vi "draw.vi"(0 "reference":refnum<class "Grid.lvclass">, 1 "graphics":refnum<class "Graphics.lvclass">, 2 "bounds":T1 {"height" format="%.2f"; "width" format="%.2f"; "y" format="%.2f"; "x" format="%.2f"}, 3 "ForceRedrawGrid":bool, 5 "error in (no error)":errorcluster) -> (14 "reference out":refnum<class "Grid.lvclass">, 19 "error out":errorcluster)   [LabVIEW 2016, in "Grid.lvclass"]
doc: "public void draw(Graphics2D g2, Rectangle2D bounds)"
uses:
  <resource>/Framework/Providers/Open_GDS/UML/Grid_class/Grid.lvclass
  <resource>/Framework/Providers/Open_GDS/UML/Graphics_class/Graphics.lvclass
  <resource>/Framework/Providers/Open_GDS/UML/General/Rectangle/Rectangle Rectangle2D.ctl
  <resource>/Framework/Providers/Open_GDS/UML/General/Point/Point Point2D.ctl
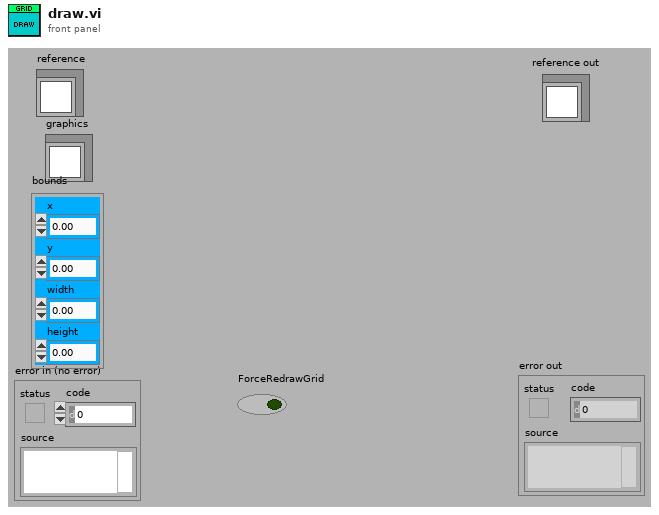
[diagram p1: front panel]
types:
  T1 = typedef "Rectangle Rectangle2D.ctl" = cluster{"x":dbl, "y":dbl, "width":dbl, "height":dbl}
  T2 = typedef "Point Point2D.ctl" = cluster{"x":dbl, "y":dbl}
  T3 = typedef "Grid.lvclass/ObjectAttributes.ctl" = cluster{"gridX":dbl, "gridY":dbl, "gridColor":u32}
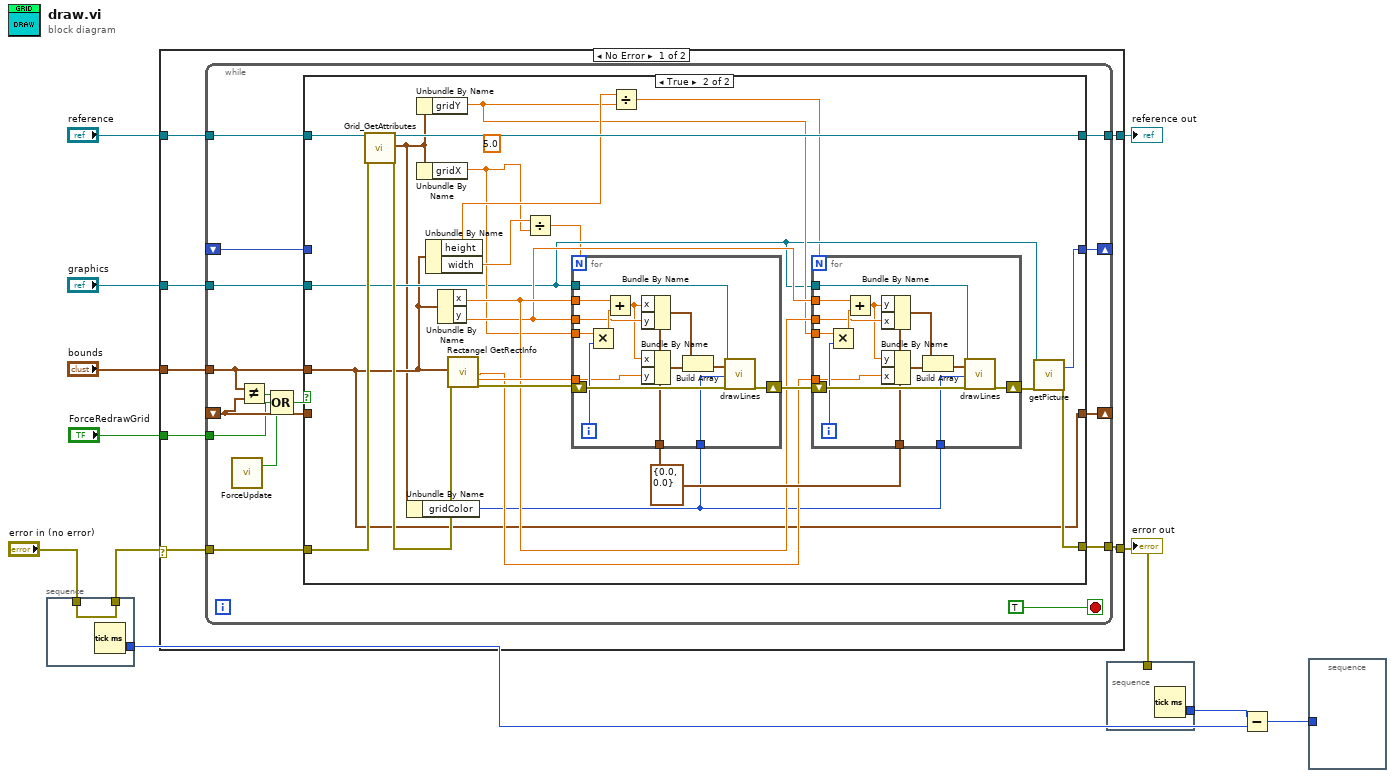
[diagram p0: block diagram]
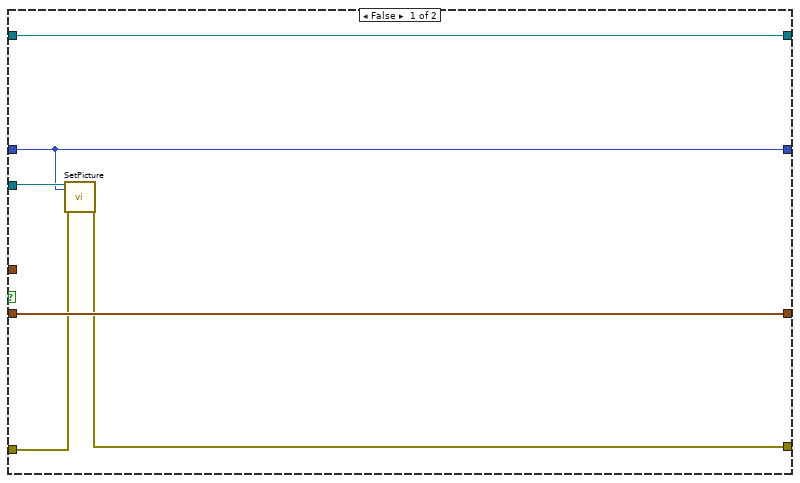
[diagram p2: hidden frame]
diagram:
  n1 = stacked-sequence {
    tunnel: [w13] -> w7
    tunnel: [w12] -> w5
    tunnel: "error in (no error)" -> [w12]
    frame #0 {
      n2 = Tick Count (ms)() -> (millisecond timer value=w13:u32)
    }
  }
  n3 = case shown="No Error" w5 {
    selector: w5 -> [w18 w96]
    tunnel: "reference" -> [w20 w97]
    tunnel: [w15 w96] -> w4
    tunnel: [w19 w97] -> w10
    tunnel: "bounds" -> [w16 _]
    tunnel: "graphics" -> [w17 _]
    tunnel: "ForceRedrawGrid" -> [w14 _]
    frame No Error {
      n4 = while {
        tunnel: w20 -> [w35]
        tunnel: [w34] -> w19
        tunnel: w18 -> [w33]
        tunnel: w17 -> [w32]
        tunnel: w16 -> [w27]
        tunnel: [w31] -> w15
        shift-right: [w29] -> _
        shift-left: _ -> [w28]
        shift-right: [w25] -> _
        shift-left: _ -> [w26]
        tunnel: w14 -> [w24]
        stop <- TRUE stop-if-true
        n5 = call <resource>:"ForceUpdate.vi"() -> ("Force"=w21:bool)  [unwired: 19 in]
        n6 = Not Equal?(x=w27, y=w28) -> (x != y?=w23:bool)
        n7 = Compound Arithmetic op=OR(w23, w24, w21) -> (w22:bool)
        n8 = case shown="True" w22 {
          tunnel: w35 -> [w40 w65]
          tunnel: [w40 w64] -> w34
          tunnel: w33 -> [w38 w63]
          tunnel: w32 -> [w39 w46]
          tunnel: w27 -> [_ w43]
          tunnel: [w37 w48] -> w31
          tunnel: [w41 w43] -> w29
          tunnel: w28 -> [w41 _]
          tunnel: w26 -> [w36 _]
          tunnel: [w36 w47] -> w25
          frame False {
            n9 = call-dynamic "SetPicture.vi"("reference"=w39, "picture"=w36, "error in (no error)"=w38) -> ("error out"=w37:errorcluster)  [unwired: 15 in, 1 out]
          }
          frame True {
            w56 = T2 {"x"=0.0, "y"=0.0} ("point2D")
            (unwired) 5.0 ("lower limit")
            n10 = call <resource>:"Grid_GetAttributes.vi"("reference in"=w65, "error in (no error)"=w63) -> ("reference out"=w64:refnum<class "Grid.lvclass">, "Data"=w42:T3, "error out"=w62:errorcluster)  [unwired: 1 in, 14 out]
            n11 = Unbundle By Name(w42) -> ("gridColor"=w50:u32)
            n12 = Unbundle By Name(w42) -> ("gridY"=w51:dbl)
            n13 = Unbundle By Name(w42) -> ("gridX"=w52:dbl)
            n14 = Unbundle By Name(w43) -> ("height"=w57:dbl, "width"=w60:dbl)
            n15 = Unbundle By Name(w43) -> ("x"=w54:dbl, "y"=w53:dbl)
            n16 = call <resource>:"Rectangel GetRectInfo.vi"("bounds"=w43, "error in (no error)"=w62) -> ("maxX"=w55:dbl, "maxY"=w59:dbl, "error out"=w61:errorcluster)  [unwired: 15 out]
            n17 = Divide(x=w60, y=w52) -> (x/y=w44:dbl)
            n18 = for {
              N: w44 -> [_]
              shift-right: [w94] -> w58
              shift-left: w61 -> [w95]
              tunnel: w46 -> [w93]
              tunnel: w56 -> [w90]
              tunnel: w52 -> [w87]
              tunnel: w54 -> [w85]
              tunnel: w53 -> [w84]
              tunnel: w59 -> [w83]
              tunnel: w50 -> [w81]
              i -> [w88]
              n19 = Multiply(x=w87, y=w88) -> (x*y=w86:dbl)
              n20 = Add(x=w85, y=w86) -> (x+y=w82:dbl)
              n21 = Bundle By Name(cluster=w90, "x"=w82, "y"=w84) -> (w89:T2)
              n22 = Bundle By Name(cluster=w90, "x"=w82, "y"=w83) -> (w91:T2)
              n23 = Build Array(w89, w91) -> (w92:T2[])
              n24 = call <resource>:"drawLines.vi"("reference"=w93, "points"=w92, "color(if not used=default color)"=w81, "error in (no error)"=w95) -> ("error out"=w94:errorcluster)  [unwired: 3 in, 12 out]
            }
            n25 = Divide(x=w57, y=w51) -> (x/y=w45:dbl)
            n26 = for {
              N: w45 -> [_]
              shift-right: [w79] -> w49
              shift-left: w58 -> [w80]
              tunnel: w46 -> [w78]
              tunnel: w56 -> [w75]
              tunnel: w51 -> [w72]
              tunnel: w53 -> [w70]
              tunnel: w54 -> [w69]
              tunnel: w55 -> [w68]
              tunnel: w50 -> [w66]
              i -> [w73]
              n27 = Multiply(x=w72, y=w73) -> (x*y=w71:dbl)
              n28 = Add(x=w70, y=w71) -> (x+y=w67:dbl)
              n29 = Bundle By Name(cluster=w75, "y"=w67, "x"=w69) -> (w74:T2)
              n30 = Bundle By Name(cluster=w75, "y"=w67, "x"=w68) -> (w76:T2)
              n31 = Build Array(w74, w76) -> (w77:T2[])
              n32 = call <resource>:"drawLines.vi"("reference"=w78, "points"=w77, "color(if not used=default color)"=w66, "error in (no error)"=w80) -> ("error out"=w79:errorcluster)  [unwired: 3 in, 12 out]
            }
            n33 = call-dynamic "getPicture.vi"("reference"=w46, "error in (no error)"=w49) -> ("picture"=w47:picture, "error out"=w48:errorcluster)  [unwired: 15 in, 1 out]
          }
        }
      }
    }
    frame Error {
    }
  }
  "reference out" <- w10
  "error out" <- w4
  n34 = stacked-sequence {
    tunnel: [w98] -> w3
    tunnel: w4 -> [_]
    frame #0 {
      n35 = Tick Count (ms)() -> (millisecond timer value=w98:u32)
    }
  }
  n36 = Subtract(x=w3, y=w7) -> (x-y=w2:u32)
  n37 = stacked-sequence {
    tunnel: w2 -> [_]
    frame #0 {
    }
  }
